vi "Set Slave Node-ID.vi"(8 "error in":errorcluster, 10 "Slave Node-ID":u8 format="%.0x", 11 "Interactor in":refnum<class "Interactor.lvclass">) -> (0 "error out":errorcluster, 3 "Interactor out":refnum<class "Interactor.lvclass">)   [LabVIEW 2024, in "Interactor.lvlib" / "Interactor.lvclass"]
uses:
  Interactor.lvclass
  Interactor.lvclass/Interactor.ctl
  Home Messages/Slave Node-ID Selected Msg/Slave Node-ID Selected Msg.lvclass/Slave Node-ID Selected Msg.ctl
  <vilib>/ActorFramework/Message Enqueuer/Message Enqueuer.lvclass/Message Enqueuer.ctl
  Home Messages/Slave Node-ID Selected Msg/Slave Node-ID Selected Msg.lvclass
  C:/Program Files/National Instruments/LabVIEW 2025/vi.lib/ActorFramework/Message/Message.lvclass
  CANopen Master/CANopen Master.lvclass
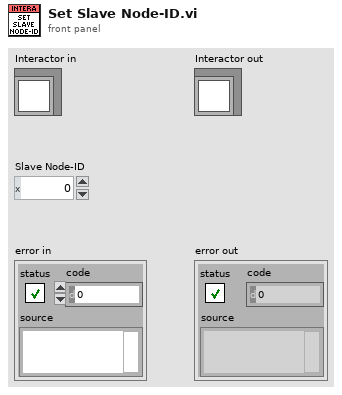
[diagram p1: front panel]
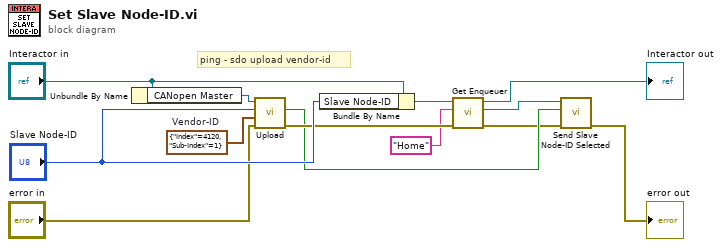
[diagram p0: block diagram]
diagram:
  w9 = cluster{"Index":u16, "Sub-Index":u8} {"Index"=4120, "Sub-Index"=1}  # Vendor-ID
  # "ping - sdo upload vendor-id"
  n1 = Unbundle By Name("Interactor in") -> ("CANopen Master"=w12:refnum<class "CANopen Master.lvclass">)
  n2 = call "Upload.vi"("error in"="error in", "Multiplexer"=w9, "Node-ID"="Slave Node-ID", "CANopen Master in"=w12) -> ("error out"=w7:errorcluster, "Success?"=w6:bool)  [unwired: 4 in, 2 out]
  n3 = Bundle By Name(cluster="Interactor in", "Slave Node-ID"="Slave Node-ID") -> (w5:refnum<class "Interactor.lvclass">)
  n4 = call "Get Enqueuer.vi"("error in"=w7, "Ident"="Home", "Interactor in"=w5) -> ("error out"=w2:errorcluster, "Enq"=w3:refnum<class "Message Enqueuer.lvclass">, "Interactor out"=→"Interactor out":refnum<class "Interactor.lvclass">)  [unwired: 6 in]
  n5 = call "Send Slave Node-ID Selected.vi"("error in (no error)"=w2, "Valid?"=w6, "Message Enqueuer"=w3) -> ("error out"=→"error out":errorcluster)  [unwired: 7 in, 1 out]
